vi "TDMS Path.vi"(8 "error in":errorcluster, 10 "Serial No":string, 11 "Socket":string="0") -> (0 "error out":errorcluster, 3 "File path":path=path "C:/Rawlogfiles/DUT/2022Jul31/092816_")   [LabVIEW 2021, in "TDMS GIP.lvlib"]
uses:
  TDMS GIP.lvlib
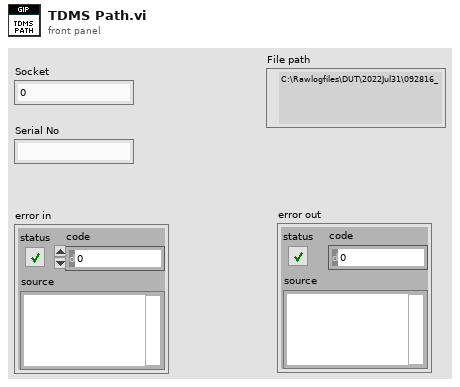
[diagram p1: front panel]
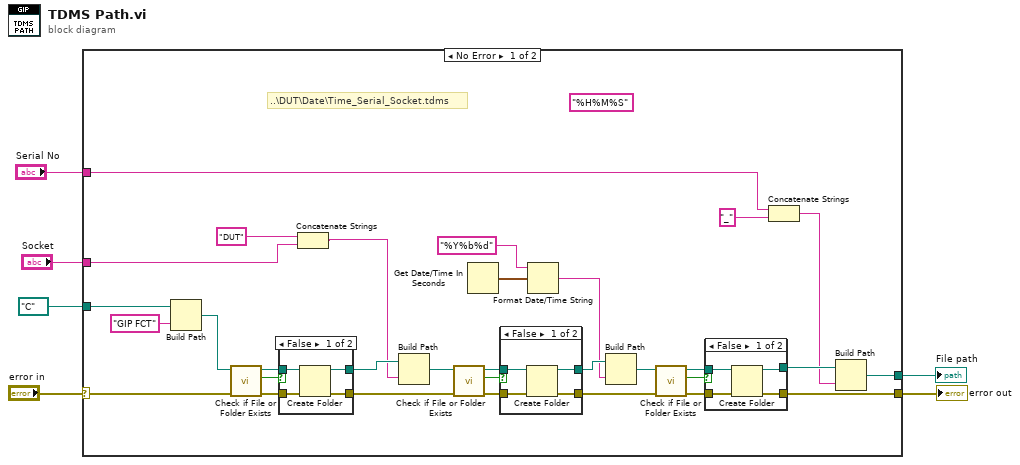
[diagram p0: block diagram]
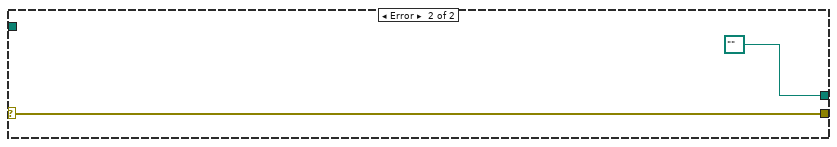
[diagram p5: hidden frame]
diagram:
  n1 = case shown="No Error" "error in" {
    selector: "error in" -> [w31 w57]
    tunnel: [w15 w57] -> w5
    tunnel: "Socket" -> [w9 _]
    tunnel: path "C:/" ("Application Directory") -> [w30 _]
    tunnel: [w13 path "" ("appended path")] -> w3
    tunnel: "Serial No" -> [w7 _]
    frame No Error {
      (unwired) "%H%M%S" ("time format string (%c)")
      # "..\\DUT\\Date\\Time_Serial_Socket.tdms"
      n2 = Build Path(base path=w30, name or relative path="GIP FCT" ("relative uri")) -> (appended path=w32:path)
      n3 = call <vilib>:"Check if File or Folder Exists.vi"("error in (no error)"=w31, "path"=w32) -> ("error out"=w34:errorcluster, "file or folder exists?"=w35:bool, "dup path"=w33:path)  [unwired: 7 in]
      n4 = case shown="False" w35 {
        tunnel: w34 -> [w53 w55]
        tunnel: [w52 w55] -> w19
        tunnel: w33 -> [w51 w54]
        tunnel: [w50 w54] -> w37
        frame False {
          n5 = Create Folder(path (use dialog)=w51, error in=w53) -> (created path=w50:path, error out=w52:errorcluster)  [unwired: 1 in, 1 out]
        }
        frame True {
        }
      }
      n6 = Concatenate Strings("DUT" ("string"), w9) -> (w8:string)
      n7 = Build Path(base path=w37, name or relative path=w8) -> (appended path=w26:path)
      n8 = call <vilib>:"Check if File or Folder Exists.vi"("error in (no error)"=w19, "path"=w26) -> ("error out"=w29:errorcluster, "file or folder exists?"=w27:bool, "dup path"=w28:path)  [unwired: 7 in]
      n9 = Get Date/Time In Seconds() -> (seconds since 1Jan1904=w18:timestamp)
      n10 = case shown="False" w27 {
        tunnel: w29 -> [w47 w49]
        tunnel: [w46 w49] -> w20
        tunnel: w28 -> [w45 w48]
        tunnel: [w44 w48] -> w25
        frame False {
          n11 = Create Folder(path (use dialog)=w45, error in=w47) -> (created path=w44:path, error out=w46:errorcluster)  [unwired: 1 in, 1 out]
        }
        frame True {
        }
      }
      n12 = Format Date/Time String(time format string (%c)="%Y%b%d", seconds (now)=w18) -> (date/time string=w16:string)  [unwired: 1 in]
      n13 = Build Path(base path=w25, name or relative path=w16) -> (appended path=w21:path)
      n14 = call <vilib>:"Check if File or Folder Exists.vi"("error in (no error)"=w20, "path"=w21) -> ("error out"=w22:errorcluster, "file or folder exists?"=w24:bool, "dup path"=w23:path)  [unwired: 7 in]
      n15 = case shown="False" w24 {
        tunnel: w22 -> [w41 w43]
        tunnel: [w40 w43] -> w15
        tunnel: w23 -> [w39 w42]
        tunnel: [w38 w42] -> w14
        frame False {
          n16 = Create Folder(path (use dialog)=w39, error in=w41) -> (created path=w38:path, error out=w40:errorcluster)  [unwired: 1 in, 1 out]
        }
        frame True {
        }
      }
      n17 = Concatenate Strings(w7, "_" ("regular expression")) -> (w12:string)
      n18 = Build Path(base path=w14, name or relative path=w12) -> (appended path=w13:path)
    }
    frame Error {
    }
  }
  "error out" <- w5
  "File path" <- w3
